vi "play_AFM_TF.vi"() -> ()   [LabVIEW 2015]
uses:
  controls/ControlParams_TF.ctl
  <vilib>/Analysis/Matrix/Datatypes/RealMatrix.ctl
  <vilib>/userdefined/High Color/nirio_resource_hc.ctl
  <vilib>/Utility/file.llb/Read From Spreadsheet File (DBL).vi
  <vilib>/Analysis/Matrix/Numeric/Conversions/Matrix To Array - RM.vi
  <vilib>/FPGAPlugInAG/cRIO-9082/niLvFpga_Open_cRIO-9082.vi
  <vilib>/rvi/interface/common/dynamic/niFpgaDynamicAddResources.vi
  <vilib>/FPGAPlugInAG/Dynamic/niLvFpga_Reset_Dynamic.vi
  <vilib>/rvi/interface/common/niFpgaWaitOnOcc.vi
  <vilib>/Utility/error.llb/Error Cluster From Error Code.vi
  <vilib>/rvi/errors/niLvFpgaAdjustHostInterfaceError.vi
  <vilib>/FPGAPlugInAG/Dynamic/niLvFpga_Run_Dynamic.vi
  <vilib>/Utility/file.llb/Write To Spreadsheet File (DBL).vi
  <vilib>/FPGAPlugInAG/Dynamic/niLvFpga_Close_Dynamic.vi
  <vilib>/rvi/interface/nirviOpenFPGA/nirviOpenFPGA.xnode
  FPGA Bitfiles/AFMsssinglematri_FPGATargetSPARTA_AFMsscontrolTF_UpMICpvpCQI.lvbitx
  <vilib>/rvi/interface/nirviMethod/nirviMethod.xnode
  <vilib>/rvi/interface/nirviReadWriteControl/nirviReadWriteControl.xnode
  <vilib>/rvi/interface/nirviCloseFPGA/nirviCloseFPGA.xnode
  <vilib>/FPGAPlugInAG/Dynamic/niLvFpga_ConfigureFifo_Dynamic.vi
  <vilib>/rvi/errors/niLvFpgaMergeErrorWithErrorCode.vi
  <vilib>/rvi/interface/Simulation/niFpgaSimulationCallBeginRW.vi
  <vilib>/FPGAPlugInAG/Dynamic/niLvFpga_ReadFifo_Dynamic.vi
  <vilib>/Analysis/Matrix/NI_Matrix.lvlib
  NiFpgaLv.dll
  <vilib>/FPGAPlugInAG/Dynamic/niLvFpga_WriteFifo_Dynamic.vi
panel:
  in  "ff_on":bool
  in  "TF ff Order":u8
  in  "den_ff":T1
  in  "num_ff":T1
  in  "den":T1
  in  "num":T1
  out "Waveform Graph":dbl[](graph)
  in  "TF Order":u8
  in  "TsTicks":u32
  in  "ControlParams":T2={"Umax "=0.0, "ymax"=0.0, "TsTicks"=0, "num"=[0.0, 0.0, 0.0, 0.0, 0.0, 0.0, 0.0, 0.0, 0.0], "den"=[0.0, 0.0, 0.0, 0.0, 0.0, 0.0, 0.0, 0.0, 0.0], "TF Order"=0, "num_ff"=[0.0, 0.0, 0.0, 0.0, 0.0, 0.0, 0.0, 0.0, 0.0], "den_ff"=[0.0, 0.0, 0.0, 0.0, 0.0, 0.0, 0.0, 0.0, 0.0], "TF_ff_order "=0, "ff_on"=FALSE}
  out "yk":sgl
  out "elements left":i32=1
  in  "reference traj path":path=path "C:/Users/arnold/Documents/MATLAB/AFM_SS/data/ref_traj_track.csv"
  in  "outputData BOTH":path=path "C:/Users/arnold/Documents/MATLAB/AFM_SS/data/exp01outputBOTH.csv"
  out "x+1":i32
  in  "SettleTicks":i32=10
  out "y iter":i32
  out "size(s)":i32
  in  "Iters":i32=25
  in  "ymax":dbl=4.0 format="%#_13g"
  in  "umax":dbl=1.0 format="%#_13g"
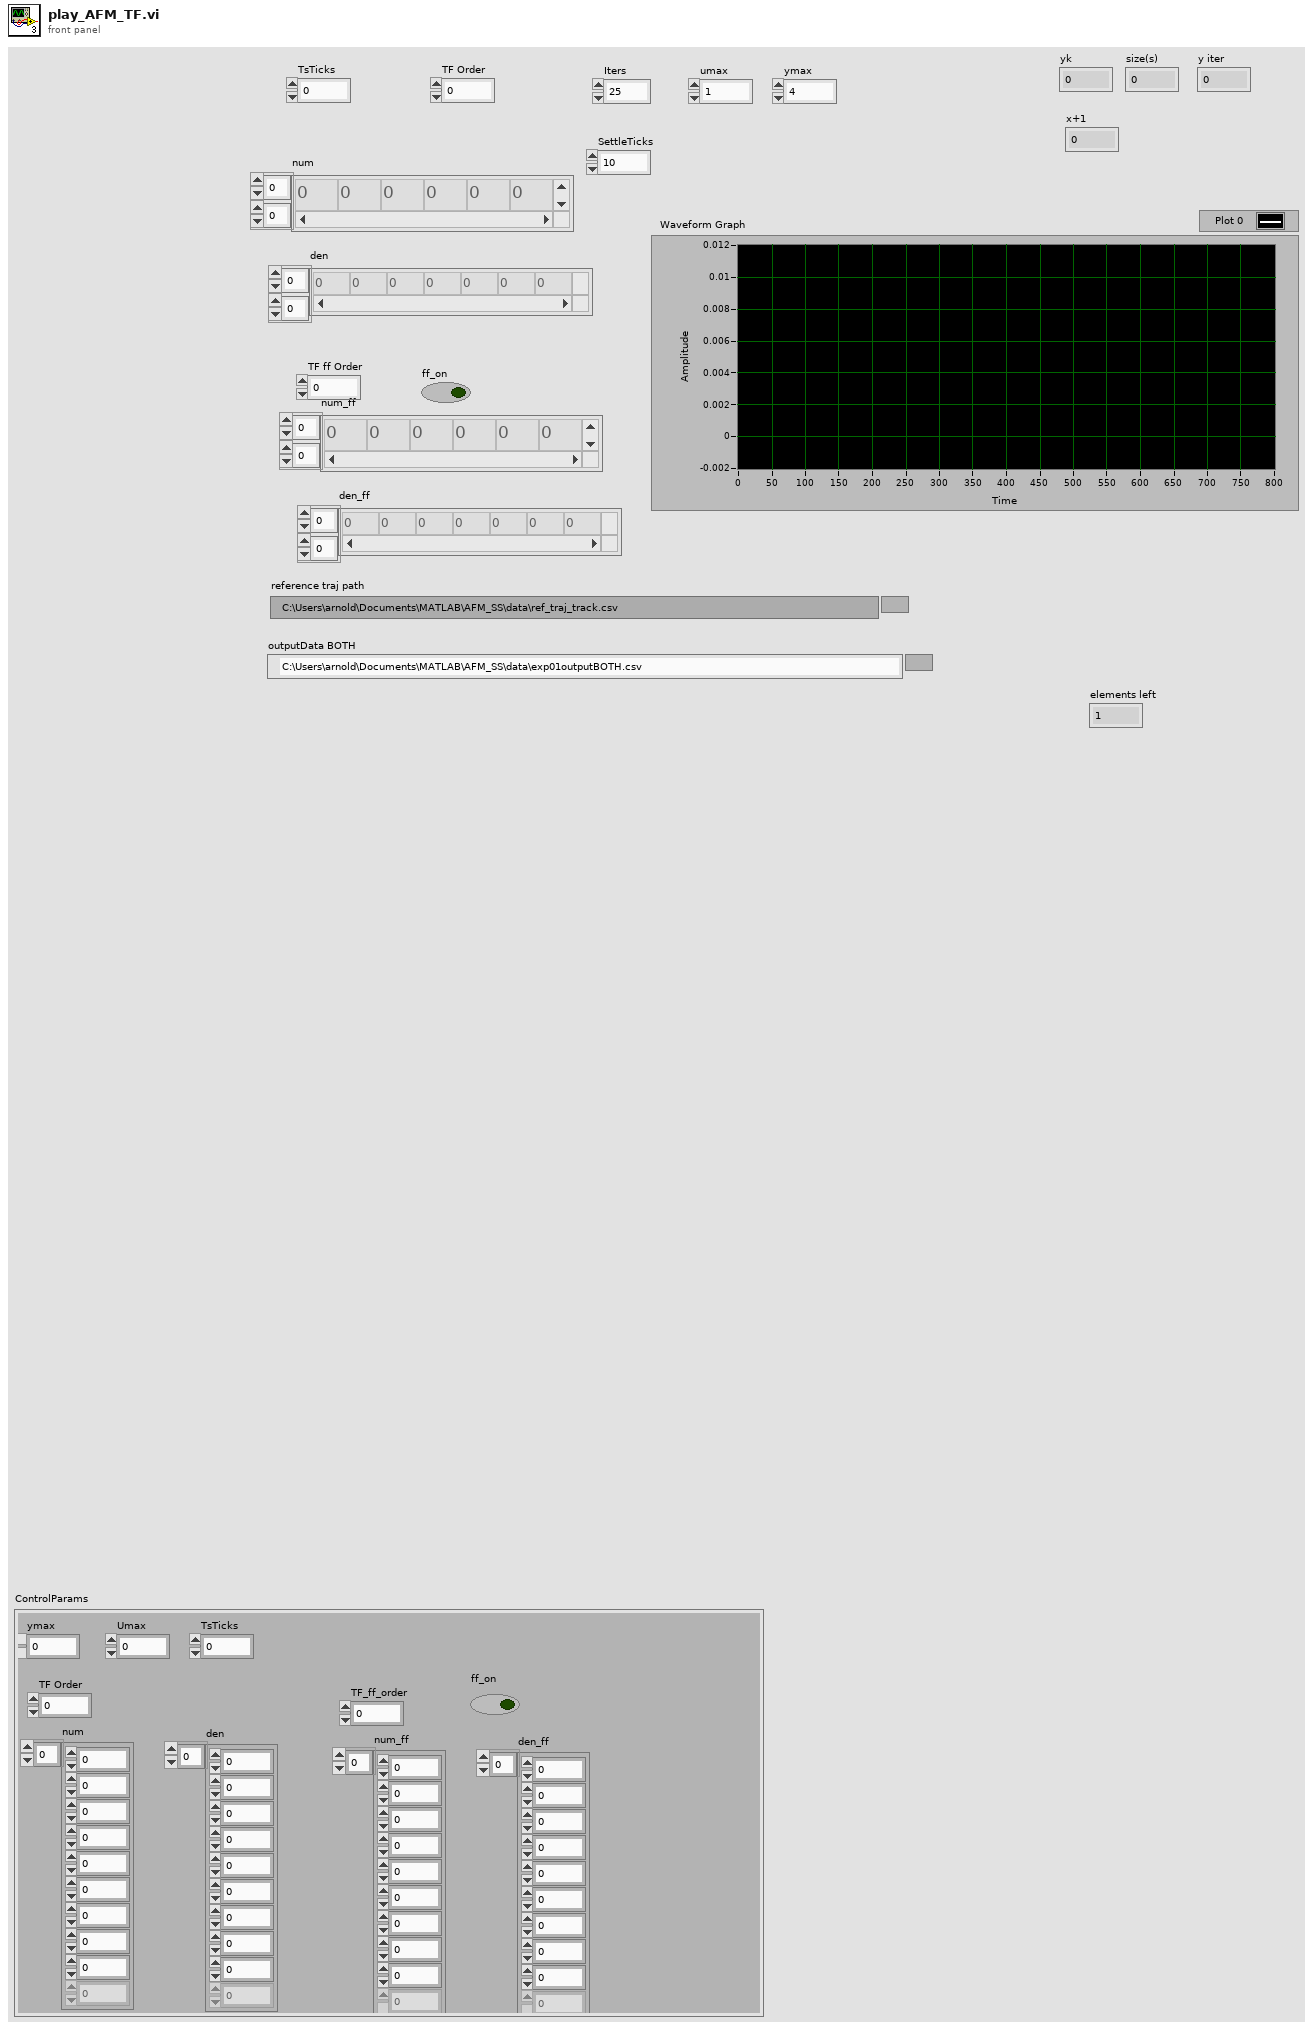
[diagram p1: front panel]
types:
  T1 = typedef "NI_Matrix.lvlib/RealMatrix.ctl" = dbl[][]
  T2 = typedef "ControlParams_TF.ctl" = cluster{"Umax ":sgl, "ymax":sgl, "TsTicks":u32, "num":sgl[], "den":sgl[], "TF Order":u8, "num_ff":sgl[], "den_ff":sgl[], "TF_ff_order ":u8, "ff_on":bool}
  T3 = typedef "nirio_resource_hc.ctl" = tag
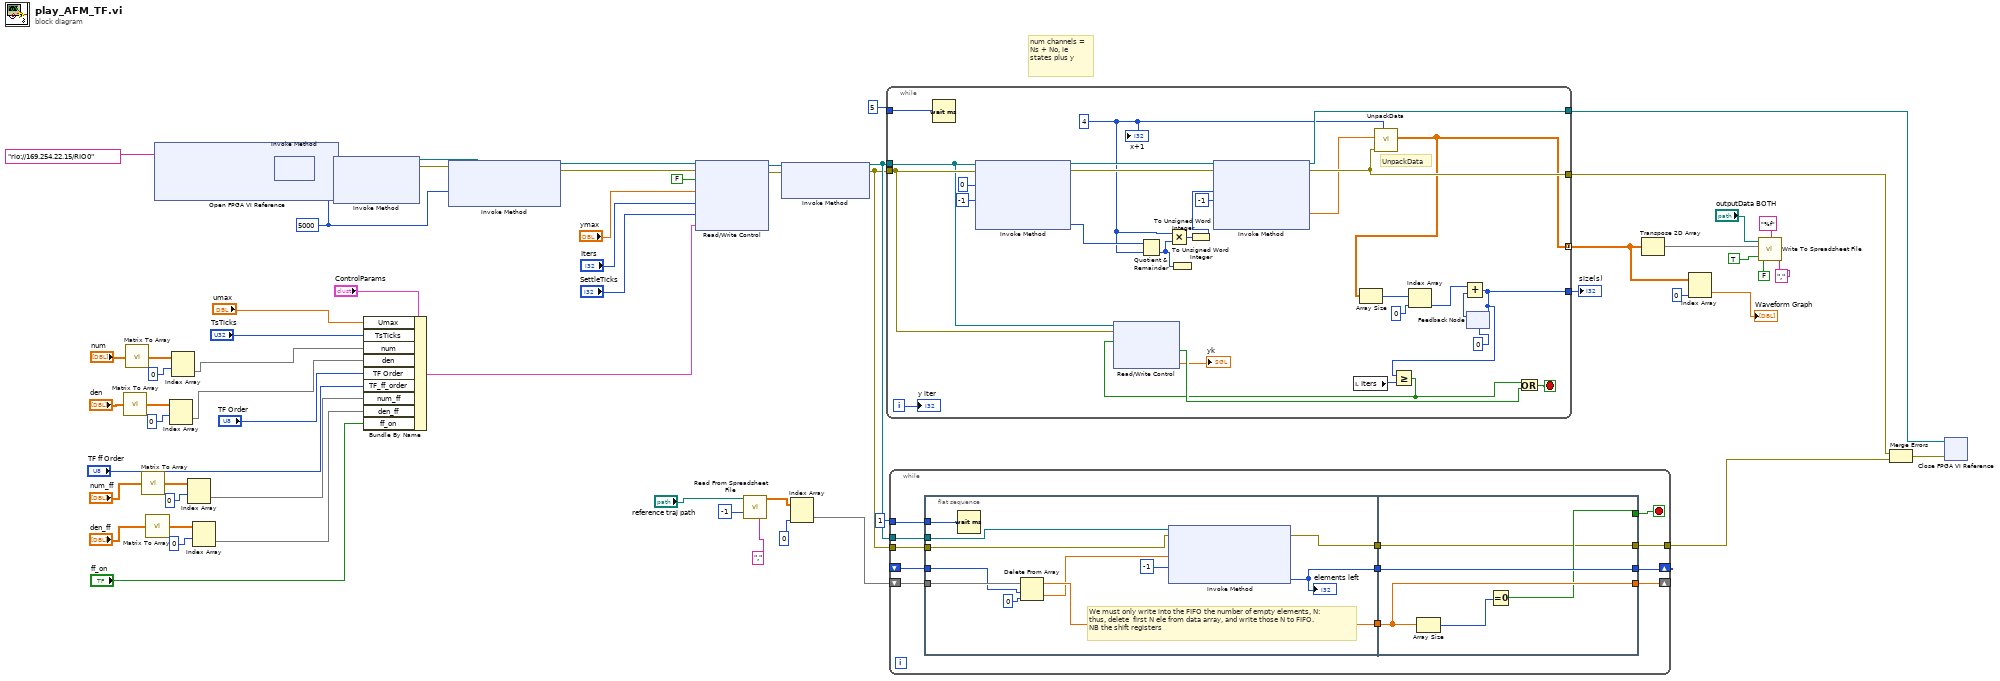
[diagram p0: block diagram]
diagram:
  w55 = 5000
  # "num channels = Ns + No, ie states plus y"
  n1 = call-poly <vilib>:"Matrix To Array.vi"("Real Matrix"="den") -> ("Real 2D Array"=w14:dbl[][])
  n2 = call-poly <vilib>:"Matrix To Array.vi"("Real Matrix"="num") -> ("Real 2D Array"=w18:dbl[][])
  n3 = call-poly <vilib>:"Matrix To Array.vi"("Real Matrix"="num_ff") -> ("Real 2D Array"=w10:dbl[][])
  n4 = call-poly <vilib>:"Matrix To Array.vi"("Real Matrix"="den_ff") -> ("Real 2D Array"=w8:dbl[][])
  n5 = xnode "Open FPGA VI Reference"("resource name"=T3 "rio://169.254.22.15/RIO0") -> ("FPGA VI Reference Out"=w54:refnum<k20>, "error out"=w53:errorcluster)  [unwired: 1 in]
  n6 = Index Array(array=w14, index (row)=0 ("disabled index (col)")) -> (element=w12:dbl[])  [unwired: 1 in]
  n7 = Index Array(array=w18, index (row)=0 ("disabled index (col)")) -> (element=w16:dbl[])  [unwired: 1 in]
  n8 = Index Array(array=w10, index (row)=0 ("disabled index (col)")) -> (element=w4:dbl[])  [unwired: 1 in]
  n9 = Index Array(array=w8, index (row)=0 ("disabled index (col)")) -> (element=w3:dbl[])  [unwired: 1 in]
  n10 = xnode "Invoke Method"("FPGA VI Reference In"=w54, "error in"=w53) -> ("FPGA VI Reference Out"=w25:refnum<k20>, "error out"=w24:errorcluster)
  n11 = xnode "Invoke Method"("FPGA VI Reference In"=w25, "error in"=w24, "Requested Depth"=w55) -> ("FPGA VI Reference Out"=w32:refnum<k20>, "error out"=w33:errorcluster)  [unwired: 1 out]
  n12 = Bundle By Name(cluster="ControlParams", "Umax"="umax", "TsTicks"="TsTicks", "num"=w16, "den"=w12, "TF Order"="TF Order", "TF_ff_order"="TF ff Order", "num_ff"=w4, "den_ff"=w3, "ff_on"="ff_on") -> (w1:T2)
  n13 = xnode "Invoke Method"("FPGA VI Reference In"=w32, "error in"=w33, "Requested Depth"=w55) -> ("FPGA VI Reference Out"=w57:refnum<k20>, "error out"=w56:errorcluster)  [unwired: 1 out]
  n14 = xnode "Read/Write Control"("FPGA VI Reference In"=w57, "error in"=w56, "Abort"=FALSE, "ymax"="ymax", "iters"="Iters", "Settle Ticks"="SettleTicks", "ControlParams"=w1) -> ("FPGA VI Reference Out"=w28:refnum<k20>, "error out"=w27:errorcluster)
  n15 = call-poly <vilib>:"Read From Spreadsheet File.vi"("delimiter (\\t)"=",", "number of rows (all:-1)"=-1, "file path (dialog if empty)"="reference traj path") -> ("all rows"=w41:dbl[][])  [unwired: 4 in, 4 out]
  n16 = xnode "Invoke Method"("FPGA VI Reference In"=w28, "error in"=w27) -> ("FPGA VI Reference Out"=w36:refnum<k20>, "error out"=w35:errorcluster)  [unwired: 1 in]
  n17 = Index Array(array=w41, index (col)=0 ("dimension size")) -> (element=w39:dbl[])  [unwired: 1 in]
  n18 = while {
    tunnel: 5 -> [w92]
    tunnel: w36 -> [w72]
    tunnel: w35 -> [w73]
    tunnel: [w84] -> w38
    tunnel: [w83] -> w60
    tunnel: [w71] -> w20 mode=concatenating
    tunnel: [w69] -> w59
    i -> [w70]
    stop <- w67 stop-if-true
    w64 = u32 4 ("y")
    # "UnpackData"
    n19 = Wait (ms)(milliseconds to wait=w92) -> ()  [unwired: 1 out]
    n20 = xnode "Invoke Method"("FPGA VI Reference In"=w72, "error in"=w73, "Number of Elements"=0 ("Timeout (ms)"), "Timeout (ms)"=-1) -> ("FPGA VI Reference Out"=w88:refnum<k20>, "error out"=w89:errorcluster, "Elements Remaining"=w79:u32)  [unwired: 1 out]
    n21 = Quotient & Remainder(x=w79, y=w64) -> (floor(x/y)=w81:u32)  [unwired: 1 out]
    n22 = Multiply(x=w64, y=w81) -> (x*y=w86:u32)
    n23 = To Unsigned Word Integer(number=w81) -> ()  [unwired: 1 out]
    n24 = To Unsigned Word Integer(number=w86) -> (unsigned 16bit integer=w82:u16)
    n25 = xnode "Invoke Method"("FPGA VI Reference In"=w88, "error in"=w89, "Number of Elements"=w82, "Timeout (ms)"=-1) -> ("FPGA VI Reference Out"=w83:refnum<k20>, "error out"=w84:errorcluster, "Data"=w78:sgl[])  [unwired: 1 out]
    n26 = local read "Iters"() -> (w80:i32)
    n27 = call "UnpackData.vi"("NumChannels"=w64, "error In"=w84, "1D Data In"=w78) -> ("2D Data Out"=w71:dbl[][])  [unwired: 7 in, 1 out]
    n28 = Array Size(array=w71) -> (size(s)=w77:i32[])
    n29 = Index Array(array=w77, index=0) -> (element=w75:i32)
    n30 = feedback #1(0) -> (w76:i32)
    n31 = Add(x=w75, y=w76) -> (x+y=w69:i32)
    n32 = Greater Or Equal?(x=w69, y=w80) -> (x >= y?=w65:bool)
    n33 = xnode "Read/Write Control"("FPGA VI Reference In"=w72, "error in"=w73, "Abort"=w65) -> ("Unstable Traj"=w68:bool, "yref_k"=→"yk":sgl)  [unwired: 2 out]
    n34 = feedback-in #1(w69) -> ()
    n35 = Or(x=w65, y=w68) -> (x .or. y?=w67:bool)
    "y iter" <- w70
    "x+1" <- w64
  }
  "size(s)" <- w59
  n36 = while {
    tunnel: [w102] -> w31
    tunnel: 1 -> [w104]
    shift-right: [w97] -> _
    shift-left: _ -> [w101]
    shift-right: [w95] -> _
    shift-left: w39 -> [w103]
    tunnel: w36 -> [w94]
    tunnel: w35 -> [w93]
    stop <- w98 stop-if-true
    n37 = flat-sequence {
      tunnel: w104 -> [w115]
      tunnel: w103 -> [w110]
      tunnel: w101 -> [w106]
      tunnel: [w113] -> w100
      tunnel: [w111] -> w99
      tunnel: [w112] -> w96
      tunnel: w94 -> [w108]
      tunnel: w93 -> [w107]
      tunnel: [w120] -> w97
      tunnel: [w116] -> w102
      tunnel: w100 -> [w116]
      tunnel: w99 -> [w120]
      tunnel: [w117] -> w98
      tunnel: w96 -> [w118]
      tunnel: [w118] -> w95
      frame #0 {
        # "We must only write into the FIFO the number of empty elements, N:\nthus, delete  first N ele from data array, and write those N to FIFO.\nNB the shift registers"
        n38 = Wait (ms)(milliseconds to wait=w115) -> ()  [unwired: 1 out]
        n39 = Delete From Array(array=w110, length=w106, index=0) -> (deleted portion=w109:dbl[], array with subset deleted=w112:dbl[])
        n40 = xnode "Invoke Method"("FPGA VI Reference In"=w108, "error in"=w107, "Data"=w109, "Timeout (ms)"=-1) -> ("error out"=w113:errorcluster, "Empty Elements Remaining"=w111:u32)  [unwired: 1 out]
        "elements left" <- w111
      }
      frame #1 {
        n41 = Array Size(array=w118) -> (size(s)=w119:i32)
        n42 = Equal To 0?(x=w119) -> (x = 0?=w117:bool)
      }
    }
  }
  n43 = Transpose 2D Array(2D array=w20) -> (transposed array=w23:dbl[][])
  n44 = Index Array(array=w20, index (col)=0 ("disabled index (col)")) -> (element=→"Waveform Graph":dbl[])  [unwired: 1 in]
  n45 = call-poly <vilib>:"Write To Spreadsheet File.vi"("delimiter (\\t)"=",", "transpose? (no:F)"=TRUE, "format (%.3f)"="%f", "append to file? (new file:F)"=FALSE, "2D data"=w23, "file path (dialog if empty)"="outputData BOTH") -> ()  [unwired: 2 in, 1 out]
  n46 = Merge Errors(w38, w31) -> (w37:errorcluster)
  n47 = xnode "Close FPGA VI Reference"("FPGA VI Reference In"=w60, "error in"=w37) -> ()  [unwired: 1 out]
